vi "F5790 Initialize.vi"(8 "error in (no error)":errorcluster, 10 "reset (F: nope)":bool, 11 "F5790 session":T1) -> (0 "error out":errorcluster, 2 "ID":string, 3 "F5790 session out":T1)   [LabVIEW 2020]
uses:
  F5790 session.ctl
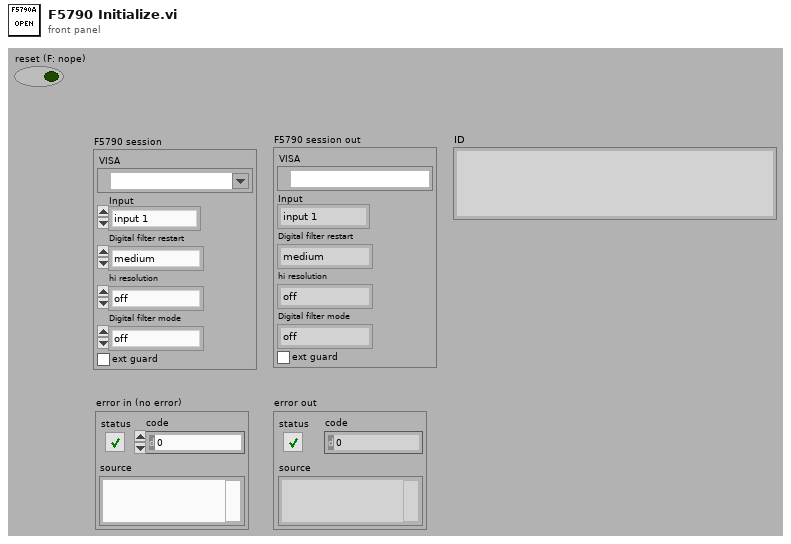
[diagram p1: front panel]
types:
  T1 = typedef "F5790 session.ctl" = cluster{"VISA":refnum<visa-resource-name>, "Input":enum16{"input 1", "input 2", "wide-band"}, "Digital filter restart":enum16{"medium", "fine", "coarse"}, "hi resolution":enum16{"off", "on"}, "Digital filter mode":enum16{"off", "fast", "medium", "slow"}, "ext guard":bool}
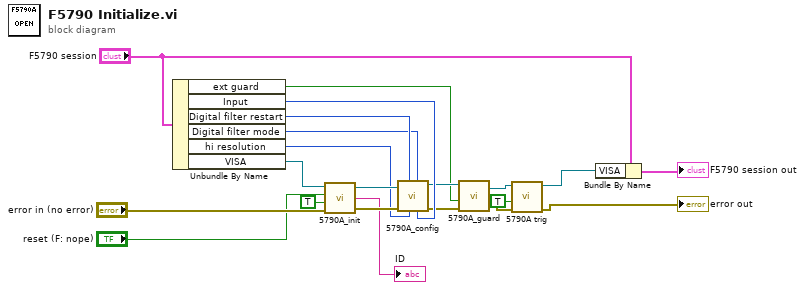
[diagram p0: block diagram]
diagram:
  n1 = Unbundle By Name("F5790 session") -> ("ext guard"=w9:bool, "Input"=w15:enum16{"input 1", "input 2", "wide-band"}, "Digital filter restart"=w14:enum16{"medium", "fine", "coarse"}, "Digital filter mode"=w13:enum16{"off", "fast", "medium", "slow"}, "hi resolution"=w12:enum16{"off", "on"}, "VISA"=w20:refnum<visa-resource-name>)
  n2 = call "5790A_init.vi"("5790A"=w20, "reset (T:yes)"="reset (F: nope)", "ID? (T:yes)"=TRUE, "error in"="error in (no error)") -> ("Session Out"=w16:refnum<visa-resource-name>, "ID"=→"ID":string, "error out"=w17:errorcluster)  [unwired: 2 in]
  n3 = call "5790A_config.vi"("Input"=w15, "Digital filter mode"=w13, "hi resolution"=w12, "Digital filter restart"=w14, "error in"=w17, "5790A"=w16) -> ("error out"=w11:errorcluster, "Session Out"=w10:refnum<visa-resource-name>)  [unwired: 4 in]
  n4 = call "5790A_guard.vi"("error in"=w11, "Guard Connection (T: external)"=w9, "5790A"=w10) -> ("error out"=w2:errorcluster, "Session Out"=w5:refnum<visa-resource-name>)  [unwired: 1 in]
  n5 = call "5790A trig.vi"("error in"=w2, "Trigger Mode (T: external)"=TRUE, "5790A"=w5) -> ("error out"=→"error out":errorcluster, "Session Out"=w3:refnum<visa-resource-name>)  [unwired: 7 in]
  n6 = Bundle By Name(cluster="F5790 session", "VISA"=w3) -> (→"F5790 session out":T1)
